vi "Cleanup_Button_Interrupt.vi"(6 "error in (no error)":errorcluster, 8 "Event Registration Refnum":refnum<event-registration>, 9 "Button Events":T1) -> (3 "Stop Local Variabl":bool)   [LabVIEW 2014]
uses:
  Interrupt/LV/Interrupt.lvlib
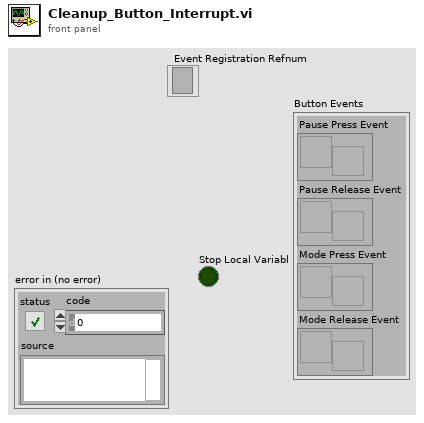
[diagram p1: front panel]
types:
  T1 = cluster{"Pause Press Event":refnum<user-event>, "Pause Release Event":refnum<user-event>, "Mode Press Event":refnum<user-event>, "Mode Release Event":refnum<user-event>}
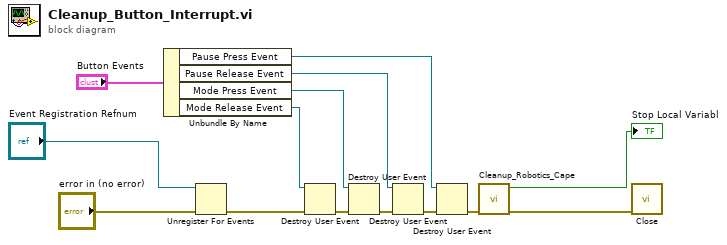
[diagram p0: block diagram]
diagram:
  n1 = Unbundle By Name("Button Events") -> ("Pause Press Event"=w4:refnum<user-event>, "Pause Release Event"=w3:refnum<user-event>, "Mode Press Event"=w2:refnum<user-event>, "Mode Release Event"=w1:refnum<user-event>)
  n2 = Unregister For Events(event registration refnum="Event Registration Refnum", error in="error in (no error)") -> (error out=w9:errorcluster)
  n3 = Destroy User Event(user event=w1, error in=w9) -> (error out=w8:errorcluster)
  n4 = Destroy User Event(user event=w2, error in=w8) -> (error out=w7:errorcluster)
  n5 = Destroy User Event(user event=w3, error in=w7) -> (error out=w6:errorcluster)
  n6 = Destroy User Event(user event=w4, error in=w6) -> (error out=w12:errorcluster)
  n7 = call "Cleanup_Robotics_Cape.vi"("error in (no error)"=w12) -> ("error out"=w13:errorcluster, "Stop Local Variabl"=→"Stop Local Variabl":bool)  [unwired: 9 in]
  n8 = call "Close.vi"("error in (no error)"=w13) -> ()  [unwired: 9 in, 2 out]
